vi "Voltaje_vrms.vi"(8 "error in (no error)":errorcluster, 11 "data":dynamicdata(waveform)) -> (0 "error out":errorcluster, 1 "Scalar":dbl, 2 "Waveform":waveform(dbl), 3 "Boolean":bool)   [LabVIEW 2019]
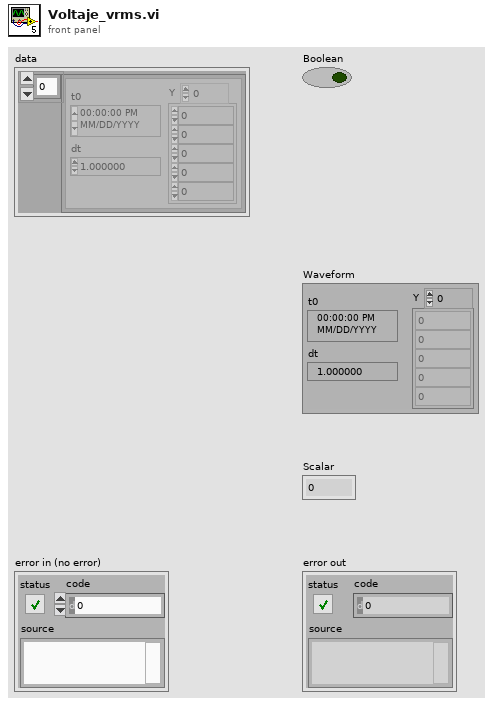
[diagram p1: front panel]
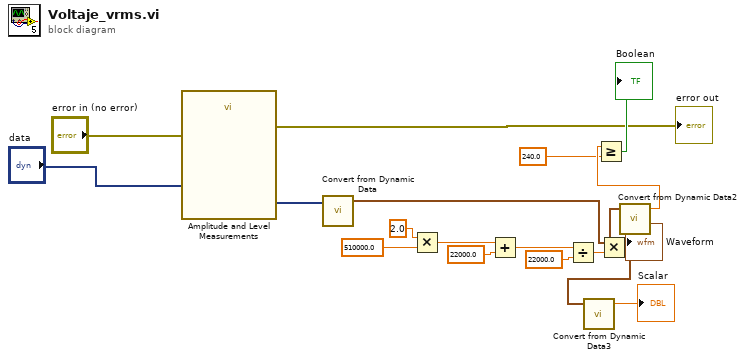
[diagram p0: block diagram]
diagram:
  n1 = call "Amplitude and Level Measurements"("Signals"="data", "error in (no error)"="error in (no error)") -> ("RMS"=w3:dynamicdata, "error out"=→"error out":errorcluster)  [unwired: 12 in]
  n2 = call "Convert from Dynamic Data"("Dynamic Data Type"=w3) -> ("Waveform"=w11:waveform(dbl))  [unwired: 3 in]
  n3 = Multiply(x=2.0, y=510000.0) -> (x*y=w6:dbl)
  n4 = Add(x=w6, y=22000.0) -> (x+y=w8:dbl)
  n5 = Divide(x=w8, y=22000.0) -> (x/y=w10:dbl)
  n6 = Multiply(x=w11, y=w10) -> (x*y=w16:waveform(dbl))
  "Waveform" <- w16
  n7 = call "Convert from Dynamic Data3"("Dynamic Data Type"=w16) -> ("Scalar"=→"Scalar":dbl)  [unwired: 3 in]
  n8 = call "Convert from Dynamic Data2"("Dynamic Data Type"=w16) -> ("Scalar"=w14:dbl)  [unwired: 3 in]
  n9 = Greater Or Equal?(x=w14, y=240.0) -> (x >= y?=→"Boolean":bool)
